vi "sub_system_IO.vi"(0 "error in 2":errorcluster caption="error in", 5 "error in":errorcluster, 11 "error in (no error)":errorcluster) -> (2 "displacement task":refnum<k21>, 4 "Parker task":refnum<k21>, 6 "acc task":refnum<k21>, 7 "displacement sample rate (S/s)":dbl=1000.0, 8 "accelerometer sample rate (S/s)":dbl, 9 "time ACC Data collection":dbl, 10 "error out":errorcluster, 13 "Accel Data":dbl[](array[numeric]), 14 "acc error":errorcluster, 15 "error out":errorcluster)   [LabVIEW 2021]
uses:
  <vilib>/DAQmx/write.llb/DAQmx Write.vi
  <vilib>/DAQmx/write.llb/DAQmx Write (Digital 1D Bool NChan 1Samp 1Line).vi
  <vilib>/DAQmx/create/channels.llb/DAQmx Create Channel (AI-Voltage-Basic).vi
  <vilib>/DAQmx/configure/timing.llb/DAQmx Timing (Sample Clock).vi
  <vilib>/DAQmx/create/channels.llb/DAQmx Create Channel (DO-Digital Output).vi
  <vilib>/DAQmx/miscellaneous.llb/DAQmx Fill In Error Info.vi
  <vilib>/DAQmx/create/channels.llb/DAQmx Create Channel (AI-Acceleration-Accelerometer).vi
  <resource>/objmgr/daqmx.rc
  <vilib>/DAQmx/read.llb/DAQmx Read (Analog 1D DBL 1Chan NSamp).vi
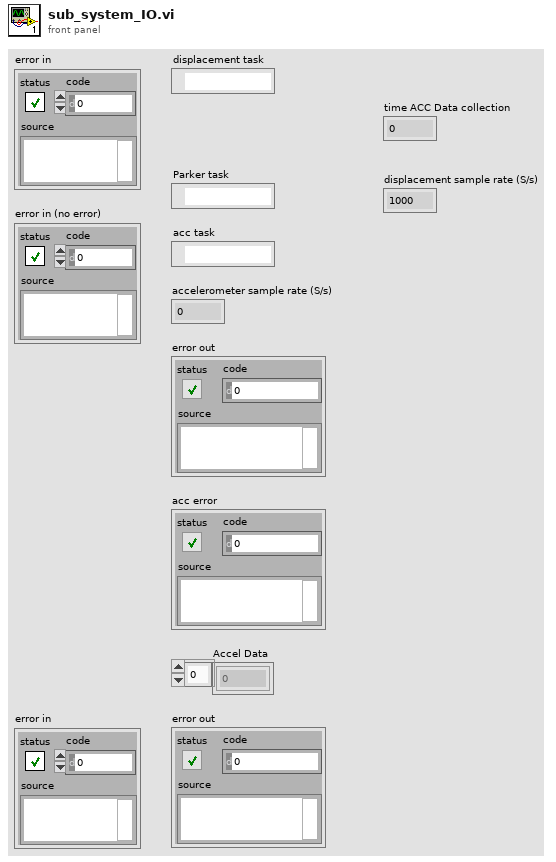
[diagram p1: front panel]
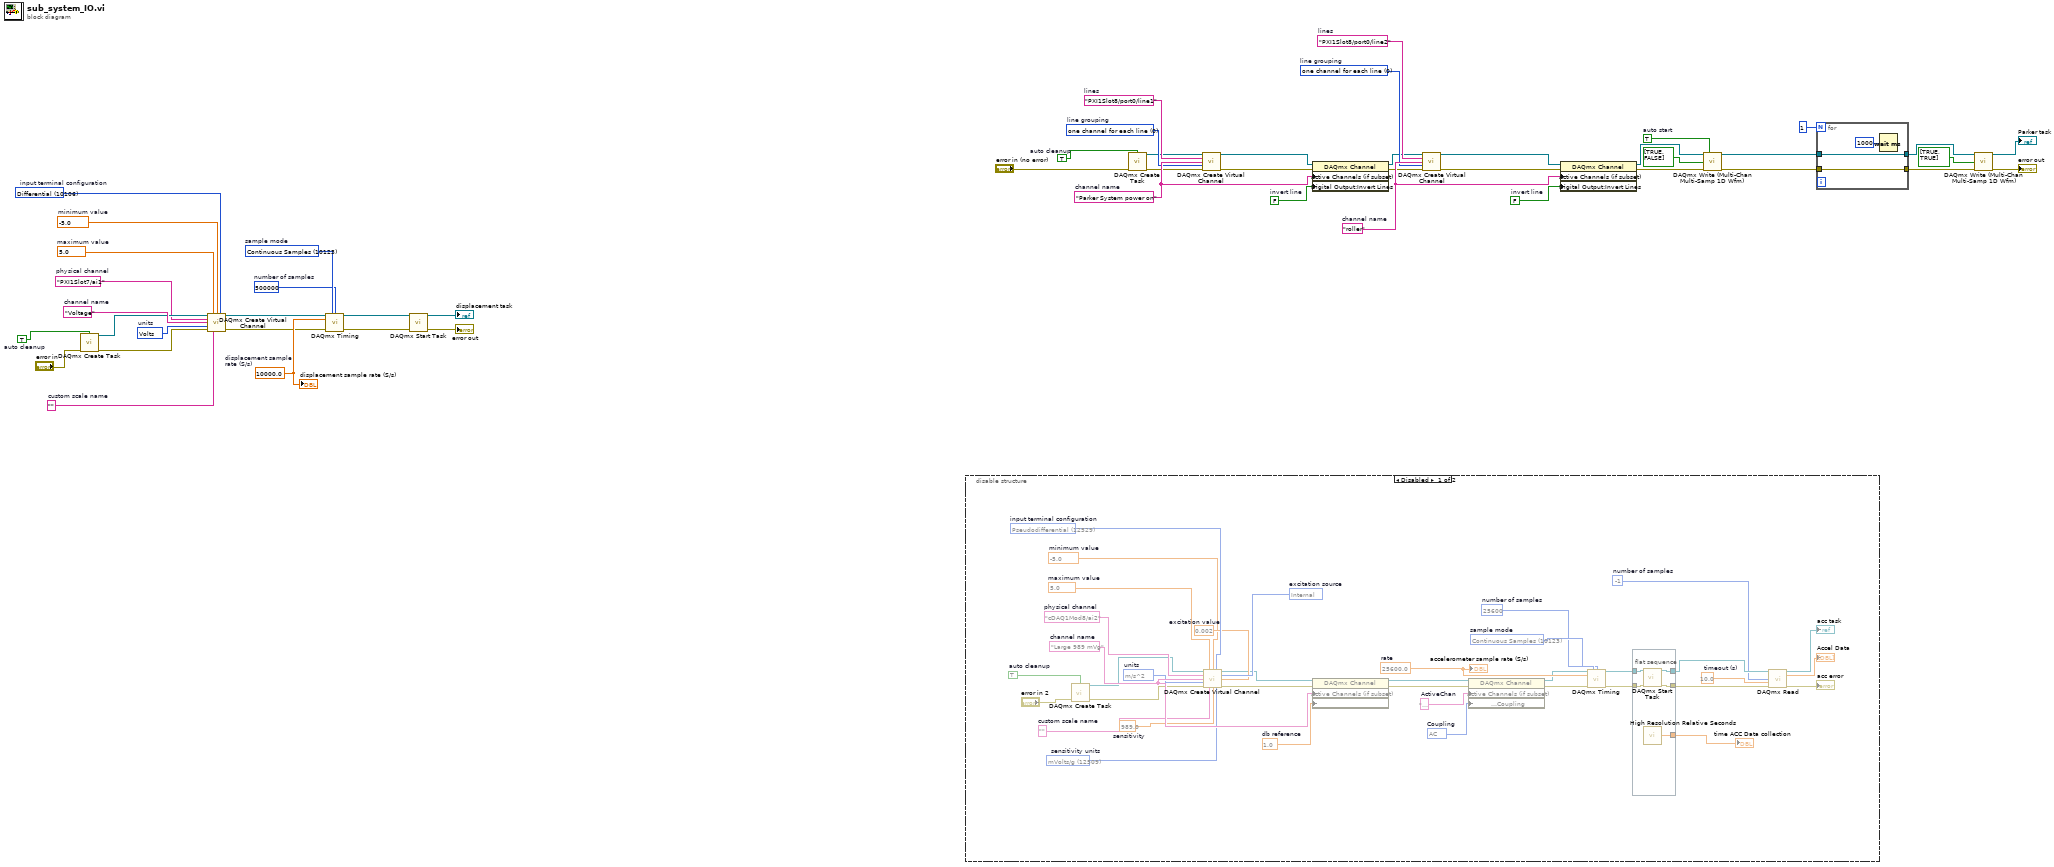
[diagram p0: block diagram]
diagram:
  w34 = FALSE  # invert line
  w31 = 0 items=["one channel for each line", "one channel for all lines"]  # line grouping
  w35 = "roller"  # channel name
  w30 = "PXI1Slot8/port0/line2"  # lines
  w27 = FALSE  # invert line
  w23 = 0 items=["one channel for each line", "one channel for all lines"]  # line grouping
  w28 = "Parker System power on"  # channel name
  w22 = "PXI1Slot8/port0/line1"  # lines
  w20 = TRUE  # auto cleanup
  w17 = TRUE  # auto start
  w16 = 10123 items=["Finite Samples"=10178, "Continuous Samples"=10123, "Hardware Timed Single Point"=12522]  # sample mode
  w15 = 500000  # number of samples
  w14 = 10000.0  # displacement sample rate (S/s)
  w12 = 10106 items=["default"=-1, "RSE"=10083, "NRSE"=10078, "Differential"=10106, "Pseudodifferential"=12529]  # input terminal configuration
  w11 = 10348 items=["Volts"=10348, "From Custom Scale"=10065]  # units
  w10 = "Voltage"  # channel name
  w8 = ""  # custom scale name
  w7 = -5.0  # minimum value
  w6 = 5.0  # maximum value
  w1 = "PXI1Slot7/ai1"  # physical channel
  w4 = TRUE  # auto cleanup
  n1 = call <vilib>:"DAQmx Create Task.vi"("auto cleanup"=w4, "error in"="error in") -> ("task out"=w5:refnum<k21>, "error out"=w3:errorcluster)  [unwired: 12 in]
  n2 = call-poly <vilib>:"DAQmx Create Virtual Channel.vi"("task in"=w5, "maximum value"=w6, "minimum value"=w7, "input terminal configuration"=w12, "physical channels"=w1, "name to assign"=w10, "units"=w11, "error in"=w3, "custom scale name"=w8) -> ("task out"=w13:refnum<k21>, "error out"=w9:errorcluster)  [unwired: 5 in]
  n3 = call-poly <vilib>:"DAQmx Timing.vi"("task/channels in"=w13, "sample mode"=w16, "samples per channel"=w15, "rate"=w14, "error in"=w9) -> ("task out"=w47:refnum<k21>, "error out"=w48:errorcluster)  [unwired: 9 in]
  n4 = call <vilib>:"DAQmx Start Task.vi"("task/channels in"=w47, "error in"=w48) -> ("task out"=→"displacement task":refnum<k21>, "error out"=→"error out":errorcluster)  [unwired: 12 in]
  n5 = disable-structure shown="Disabled" {
    frame Disabled {
      w81 = 10.0  # timeout (s)
      w80 = -1  # number of samples
      w77 = 10123 items=["Finite Samples"=10178, "Continuous Samples"=10123, "Hardware Timed Single Point"=12522]  # sample mode
      w76 = 25600  # number of samples
      w87 = 25600.0  # rate
      w72 = 10045 items=["AC"=10045, "DC"=10050, "GND"=10066]  # Coupling
      w71 = "Large 989 mVg"  # ActiveChan
      w69 = 1.0  # db reference
      w66 = 12470 items=["g"=10186, "m/s^2"=12470, "From Custom Scale"=10065]  # units
      w65 = 12529 items=["default"=-1, "RSE"=10083, "NRSE"=10078, "Differential"=10106, "Pseudodifferential"=12529]  # input terminal configuration
      w64 = 10200 items=["Internal"=10200, "External"=10167, "None"=10230]  # excitation source
      w63 = 0.002  # excitation value
      w62 = 12509 items=["mVolts/g"=12509, "Volts/g"=12510]  # sensitivity units
      w61 = 989.0  # sensitivity
      w70 = "Large 989 mVg"  # channel name
      w59 = ""  # custom scale name
      w58 = -5.0  # minimum value
      w57 = 5.0  # maximum value
      w56 = "cDAQ1Mod8/ai2"  # physical channel
      w54 = TRUE  # auto cleanup
      n6 = call <vilib>:"DAQmx Create Task.vi"("auto cleanup"=w54, "error in"="error in 2") -> ("task out"=w55:refnum<k21>, "error out"=w53:errorcluster)  [unwired: 12 in]
      n7 = call-poly <vilib>:"DAQmx Create Virtual Channel.vi"("task in"=w55, "maximum value"=w57, "minimum value"=w58, "input terminal configuration"=w65, "physical channels"=w56, "current excitation source"=w64, "name to assign"=w70, "current excitation value"=w63, "units"=w66, "error in"=w53, "custom scale name"=w59, "sensitivity"=w61, "sensitivity units"=w62) -> ("task out"=w60:refnum<k21>, "error out"=w67:errorcluster)  [unwired: 1 in]
      n8 = property class="DAQmx Channel"(reference=w60, error in=w67, "Active Channels (if subset)"=w70, "Analog Input:Acceleration:dB Reference"=w69) -> (reference out=w74:refnum<k21>, error out=w68:errorcluster)
      n9 = property class="DAQmx Channel"(reference=w74, error in=w68, "Active Channels (if subset)"=w71, "Analog Input:General Properties:Input Configuration:Coupling"=w72) -> (reference out=w75:refnum<k21>, error out=w73:errorcluster)
      n10 = call-poly <vilib>:"DAQmx Timing.vi"("task/channels in"=w75, "sample mode"=w77, "samples per channel"=w76, "rate"=w87, "error in"=w73) -> ("task out"=w78:refnum<k21>, "error out"=w79:errorcluster)  [unwired: 9 in]
      n11 = flat-sequence {
        tunnel: [w92] -> w84
        tunnel: [w91] -> w82
        tunnel: w79 -> [w90]
        tunnel: w78 -> [w89]
        tunnel: [w88] -> w51
        frame #0 {
          n12 = call <vilib>:"DAQmx Start Task.vi"("task/channels in"=w89, "error in"=w90) -> ("task out"=w92:refnum<k21>, "error out"=w91:errorcluster)  [unwired: 12 in]
          n13 = call <vilib>:"High Resolution Relative Seconds.vi"() -> ("relative seconds"=w88:dbl)
        }
      }
      n14 = call-poly <vilib>:"DAQmx Read.vi"("task/channels in"=w84, "number of samples per channel"=w80, "timeout"=w81, "error in"=w82) -> ("task out"=→"acc task":refnum<k21>, "data"=→"Accel Data":dbl[], "error out"=→"acc error":errorcluster)  [unwired: 9 in]
      "accelerometer sample rate (S/s)" <- w87
      "time ACC Data collection" <- w51
    }
    frame Enabled {
    }
  }
  n15 = call <vilib>:"DAQmx Create Task.vi"("auto cleanup"=w20, "error in"="error in (no error)") -> ("task out"=w21:refnum<k21>, "error out"=w19:errorcluster)  [unwired: 12 in]
  n16 = call-poly <vilib>:"DAQmx Create Virtual Channel.vi"("task in"=w21, "lines"=w22, "name to assign"=w28, "line grouping"=w23, "error in"=w19) -> ("task out"=w24:refnum<k21>, "error out"=w25:errorcluster)  [unwired: 9 in]
  n17 = property class="DAQmx Channel"(reference=w24, error in=w25, "Active Channels (if subset)"=w28, "Digital Output:Invert Lines"=w27) -> (reference out=w29:refnum<k21>, error out=w26:errorcluster)
  n18 = call-poly <vilib>:"DAQmx Create Virtual Channel.vi"("task in"=w29, "lines"=w30, "name to assign"=w35, "line grouping"=w31, "error in"=w26) -> ("task out"=w32:refnum<k21>, "error out"=w33:errorcluster)  [unwired: 9 in]
  n19 = property class="DAQmx Channel"(reference=w32, error in=w33, "Active Channels (if subset)"=w35, "Digital Output:Invert Lines"=w34) -> (reference out=w36:refnum<k21>, error out=w37:errorcluster)
  n20 = call-poly "DAQmx Write (Multi-Chan Multi-Samp 1D Wfm).vi"("task/channels in"=w36, "auto start"=w17, "data"=bool[] [TRUE, FALSE], "error in"=w37) -> ("task out"=w40:refnum<k21>, "error out"=w41:errorcluster)  [unwired: 9 in, 1 out]
  n21 = for {
    N: 1 -> [_]
    tunnel: [w95] -> w39
    tunnel: w40 -> [w95]
    tunnel: w41 -> [w94]
    tunnel: [w94] -> w42
    n22 = Wait (ms)(milliseconds to wait=u32 1000) -> ()  [unwired: 1 out]
  }
  n23 = call-poly "DAQmx Write (Multi-Chan Multi-Samp 1D Wfm).vi"("task/channels in"=w39, "data"=bool[] [TRUE, TRUE], "error in"=w42) -> ("task out"=→"Parker task":refnum<k21>, "error out"=→"error out":errorcluster)  [unwired: 10 in, 1 out]
  "displacement sample rate (S/s)" <- w14
